vi "Write_Data.vi"(8 "error in (no error)":errorcluster caption="entrée d'erreur (pas d'erreur)", 10 "Data_To_Write":string, 11 "Class Instrument Firebase Altyor en entrée":refnum<class "Class Instrument Database Altyor.lvclass">) -> (0 "error out":errorcluster caption="sortie d'erreur", 3 "Class Instrument Firebase Altyor en sortie":refnum<class "Class Instrument Database Altyor.lvclass">)   [LabVIEW 2020, in "Library Instrument & Equipement.lvlib" / "Library Instruments.lvlib" / "Class Instrument Database Altyor.lvclass"]
uses:
  Class Instrument Database Altyor.lvclass
  Class Instrument Database Altyor.lvclass/Class Instrument Database Altyor.ctl
  JSON API/JSON Value/Set from JSON string.vi
  JSON API/JSON Value/JSON Value.lvclass
  Database/Database Altyor/Database Altyor.lvclass
  JSON API/Variant JSON/Variant JSON.lvlib
  JSON API/Get Polymorphic/JSON GetSet.lvlib
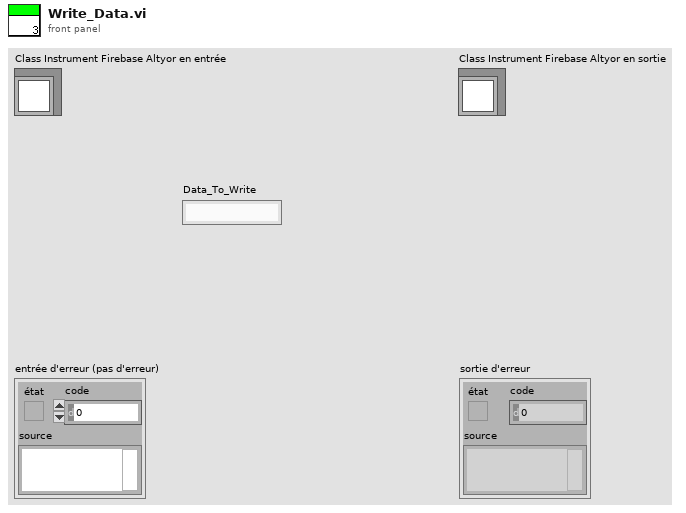
[diagram p1: front panel]
types:
  T1 = cluster{"idTest":u32, "CreationDate":string, "EndOfProduction":string, "OrderNumber":string, "Batch":string, "ProductName":string, "PartNumber":string, "SerialNumber":string, "Operator":string, "Result":string, "AdditionalInformation":string}[]
  T2 = cluster{"idTest":u32, "CreationDate":string, "EndOfProduction":string, "OrderNumber":string, "Batch":string, "ProductName":string, "PartNumber":string, "SerialNumber":string, "Operator":string, "Result":string, "AdditionalInformation":string}
  T3 = cluster{"Key_Test":u32, "idTest":u32, "MainTest":string, "Name":string, "StartOfTest":string, "EndOfTest":string, "Result":string, "LimitMax":string, "Value":string, "LimitMin":string, "Type":string}[]
  T4 = cluster{"Key_Test":u32, "idTest":u32, "MainTest":string, "Name":string, "StartOfTest":string, "EndOfTest":string, "Result":string, "LimitMax":string, "Value":string, "LimitMin":string, "Type":string}
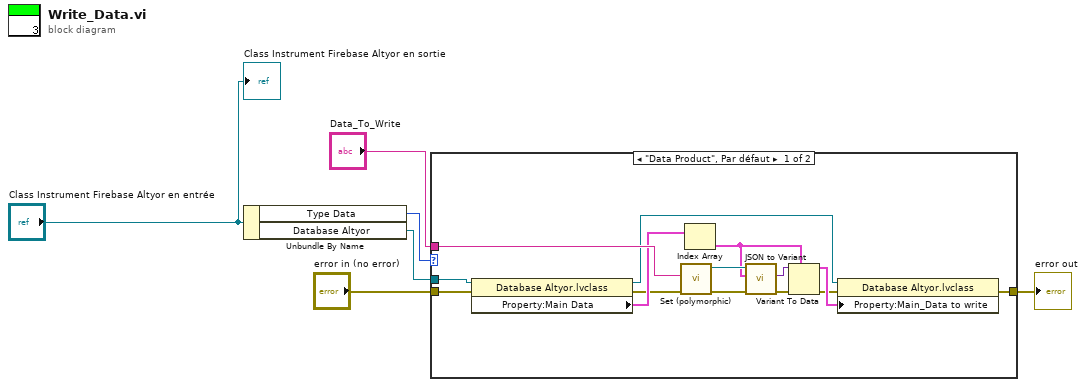
[diagram p0: block diagram]
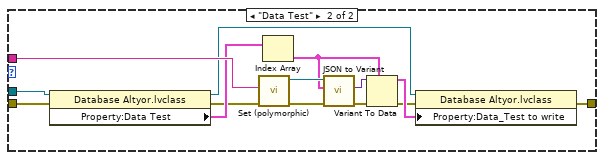
[diagram p2: hidden frame]
diagram:
  n1 = Unbundle By Name("Class Instrument Firebase Altyor en entrée") -> ("Type Data"=w6:enum16{"Data Product", "Data Test"}, "Database Altyor"=w5:refnum<class "Database Altyor.lvclass">)
  n2 = case shown="\"Data Product\", Par défaut" w6 {
    tunnel: "error in (no error)" -> [w13 w27]
    tunnel: w5 -> [w14 w28]
    tunnel: "Data_To_Write" -> [w15 w29]
    tunnel: [w20 w34] -> w1
    frame "Data Product", Default {
      n3 = property class="Database Altyor.lvclass"(reference=w14, error in=w13) -> (reference out=w12:refnum<class "Database Altyor.lvclass">, error out=w9:errorcluster, "Property:Main Data"=w11:T1)
      n4 = call-poly "Set (polymorphic).vi"("error in (no error)"=w9, "JSON stream"=w15) -> ("error out"=w17:errorcluster, "JSON Value out"=w19:refnum<class "JSON Value.lvclass">)  [unwired: 7 in, 1 out]
      n5 = Index Array(array=w11) -> (element=w7:T2)  [unwired: 1 in]
      n6 = call "JSON to Variant.vi"("error in (no error)"=w17, "Variant (Data Type)"=w7, "JSON Value"=w19) -> ("error out"=w18:errorcluster, "Variant out"=w16:variant)  [unwired: 7 in]
      n7 = Variant To Data(error in=w18, type=w7, Variant=w16) -> (data=w10:T2, error out=w8:errorcluster)
      n8 = property class="Database Altyor.lvclass"(reference=w12, error in=w8, "Property:Main_Data to write"=w10) -> (error out=w20:errorcluster)  [unwired: 1 out]
    }
    frame "Data Test" {
      n9 = property class="Database Altyor.lvclass"(reference=w28, error in=w27) -> (reference out=w26:refnum<class "Database Altyor.lvclass">, error out=w23:errorcluster, "Property:Data Test"=w25:T3)
      n10 = call-poly "Set (polymorphic).vi"("error in (no error)"=w23, "JSON stream"=w29) -> ("error out"=w31:errorcluster, "JSON Value out"=w33:refnum<class "JSON Value.lvclass">)  [unwired: 7 in, 1 out]
      n11 = Index Array(array=w25) -> (element=w21:T4)  [unwired: 1 in]
      n12 = call "JSON to Variant.vi"("error in (no error)"=w31, "Variant (Data Type)"=w21, "JSON Value"=w33) -> ("error out"=w32:errorcluster, "Variant out"=w30:variant)  [unwired: 7 in]
      n13 = Variant To Data(error in=w32, type=w21, Variant=w30) -> (data=w24:T4, error out=w22:errorcluster)
      n14 = property class="Database Altyor.lvclass"(reference=w26, error in=w22, "Property:Data_Test to write"=w24) -> (error out=w34:errorcluster)  [unwired: 1 out]
    }
  }
  "error out" <- w1
  "Class Instrument Firebase Altyor en sortie" <- "Class Instrument Firebase Altyor en entrée"
